vi "RT Loop - DL.vi"(11 "Message Queue":refnum<queue>) -> ()   [LabVIEW 2018]
doc: "This Control Loop VI performs control calculations of diverter line (DL) rotation."
uses:
  Support/Message Queue/Message Cluster.ctl
  Support/Message Queue/Message.ctl
  <vilib>/Platform/TimedLoop/XDataNode/timing_clust.ctl
  <vilib>/Platform/TimedLoop/XDataNode/nitl_modes.ctl
  <vilib>/Platform/TimedLoop/XDataNode/wakeup.ctl
  Controls/DL State.ctl
  <vilib>/Platform/TimedLoop/XDataNode/loadnilvce.vi
  <vilib>/Platform/TimedLoop/XDataNode/XDataNode.xnode
  <vilib>/Platform/TimedLoop/XDataNode/XDNodeRunTimeDep.lvlib
  support/Message Queue/Message Queue.lvlib
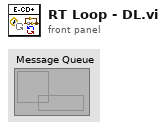
[diagram p1: front panel]
types:
  T1 = typedef "XDNodeRunTimeDep.lvlib/timing_clust.ctl" = cluster{"Expected End [f-1]":u64, "Actual End [f-1]":u64, "Finished Late? [f-1]":bool, "Expected End [i-1]":u64, "Actual End [i-1]":u64, "Finished Late? [i-1]":bool, "Expected Start [i]":u64, "Actual Start [i]":u64, "Expected Start [f]":u64, "Actual Start [f]":u64, "Source Name":string, "Structure Name":string, "Period":i64, "Deadline":i64, "Offset":i64, "Start":i64, "Priority":i32, "Timeout":i32, "Mode":T2, "Wakeup Reason":T3, "Error":errorcluster, "Source Type":string, "Secondary Source Type":string, "Global End Time":u64, "Global Start Time":u64, "Frame Duration":u64, "Iteration Duration":u64, "Assigned CPU":i32, "I/O Scan Engine Mode":u32}
  T2 = typedef "XDNodeRunTimeDep.lvlib/nitl_modes.ctl" = enum32{"No Change", "Process missed periods, maintain original phase", "Discard missed periods, maintain original phase", "Process missed periods, ignore original phase", "Discard missed periods, ignore original phase"}
  T3 = typedef "XDNodeRunTimeDep.lvlib/wakeup.ctl" = enum32{"Normal", "Aborted", "Asynchronous wakeup", "Timing source error", "Timed loop error", "Timeout"}
  T4 = typedef "DL State.ctl" = enum16{"DL STOP", "DL ROTATE CW", "DL ROTATE CCW", "SV-3 DL CW TRUE", "SV-3 DL CW FALSE", "SV-3 DL CCW TRUE", "SV-3 DL CCW FALSE"}
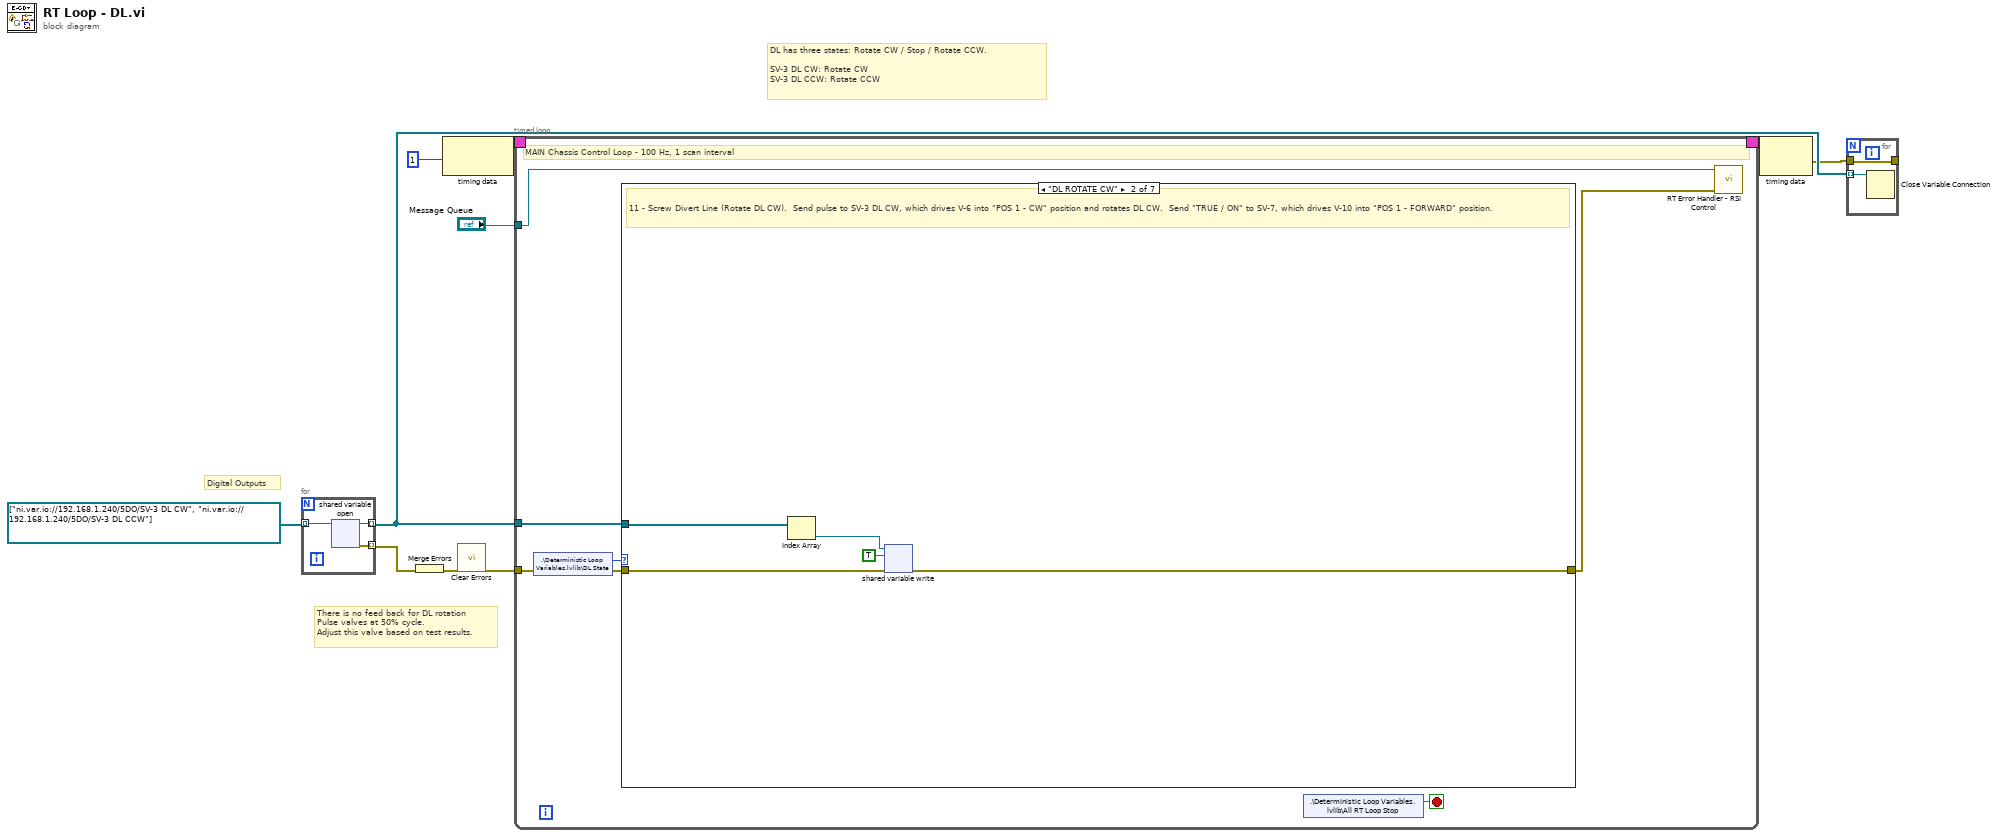
[diagram p0: block diagram]
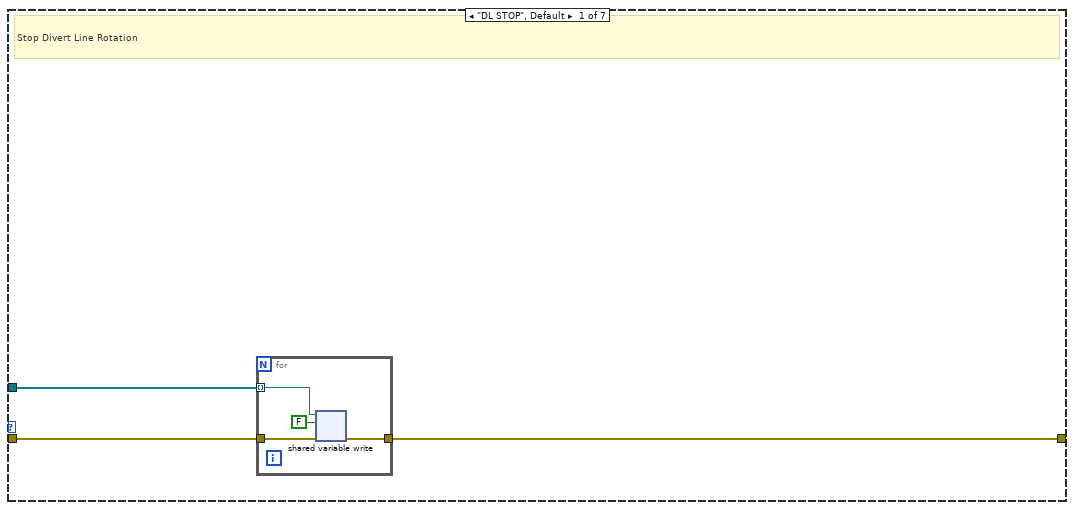
[diagram p2: hidden frame]
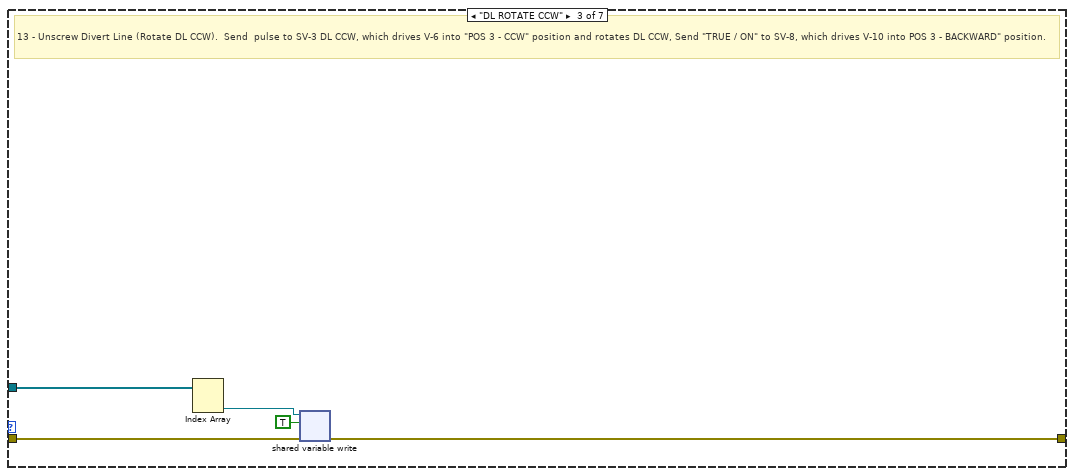
[diagram p3: hidden frame]
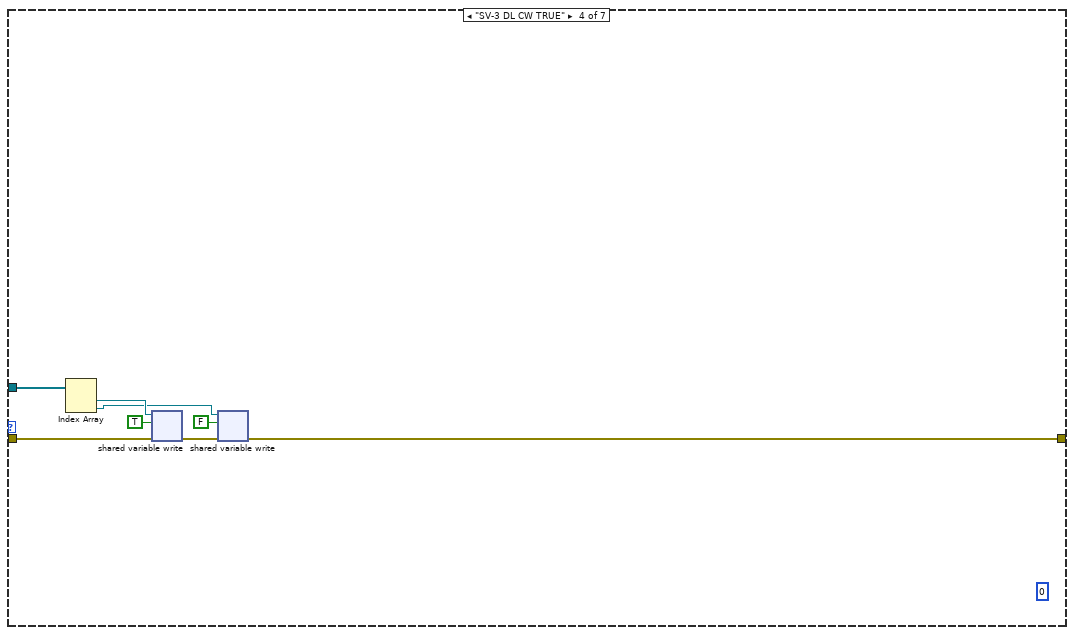
[diagram p4: hidden frame]
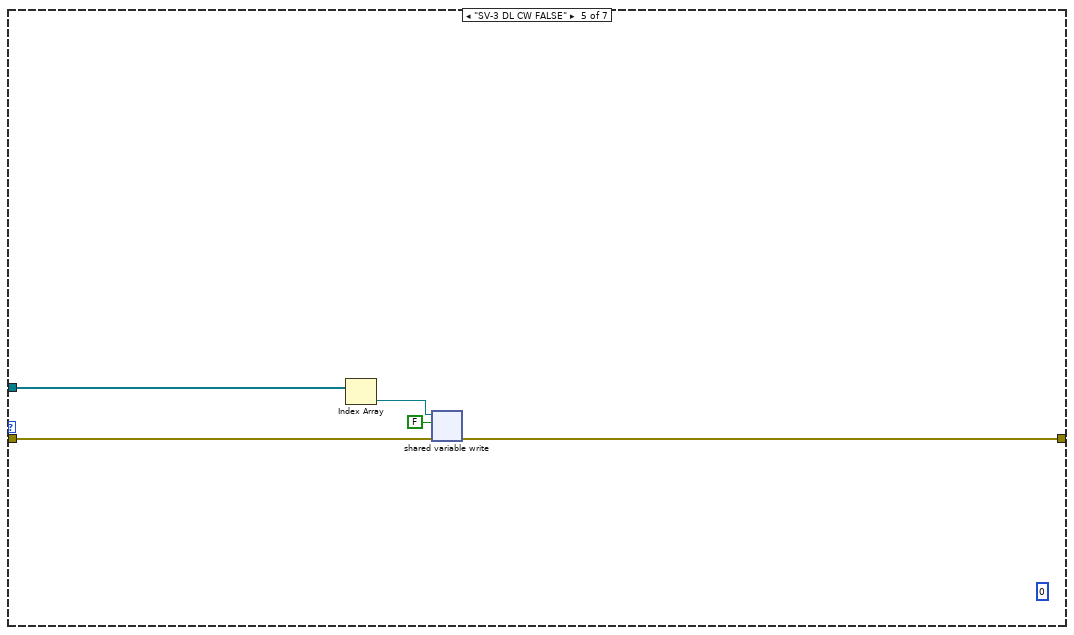
[diagram p5: hidden frame]
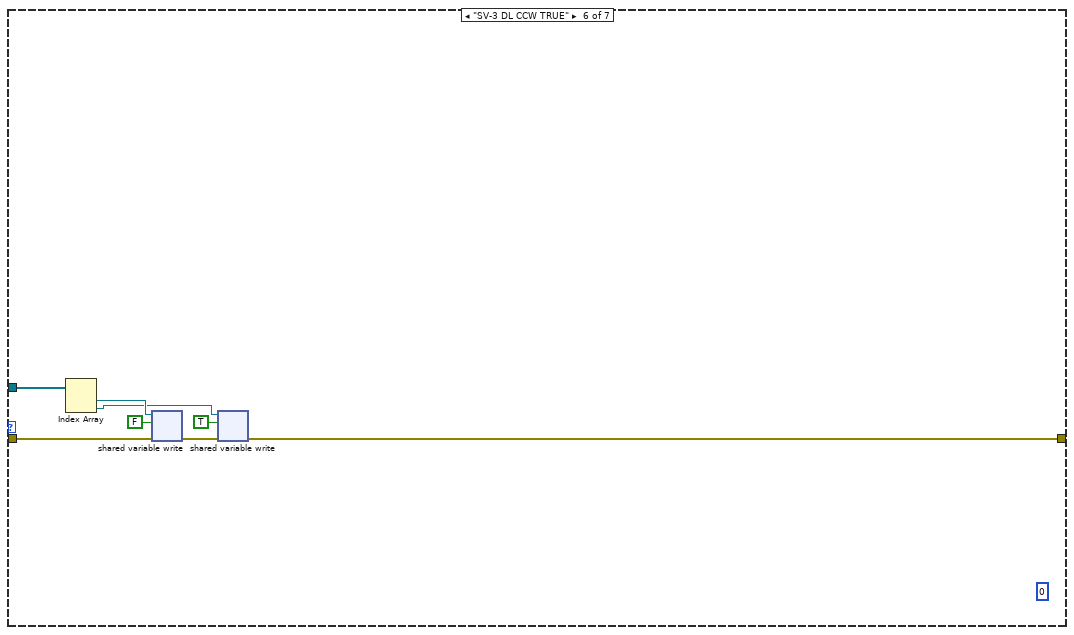
[diagram p6: hidden frame]
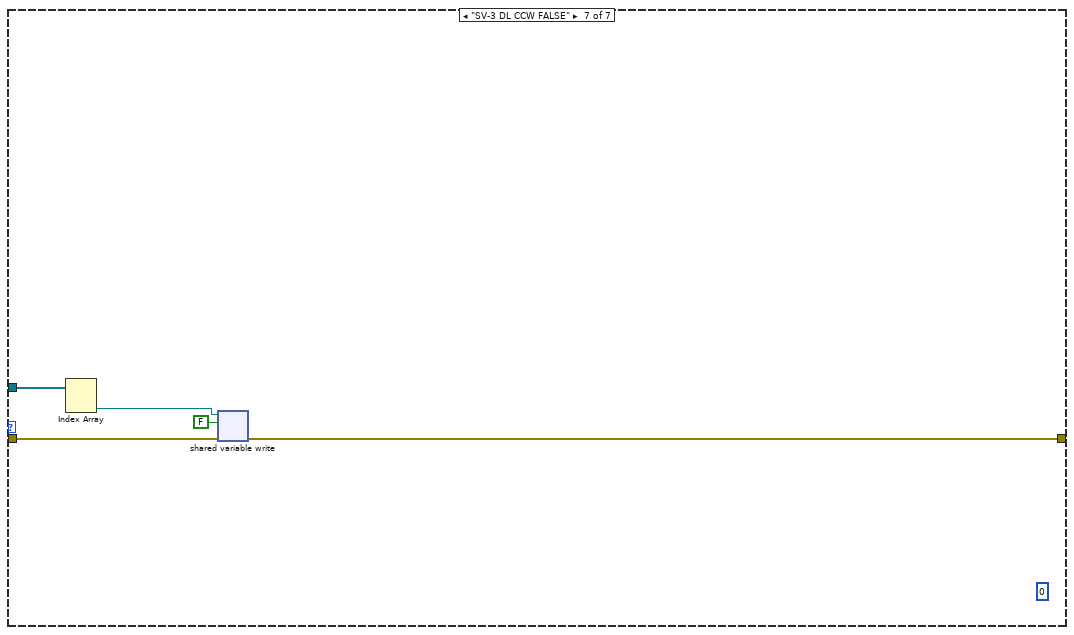
[diagram p7: hidden frame]
diagram:
  # "There is no feed back for DL rotation\nPulse valves at 50% cycle. \nAdjust this valve based on test results."
  # "Digital Outputs"
  # "DL has three states: Rotate CW / Stop / Rotate CCW.\n\nSV-3 DL CW: Rotate CW\nSV-3 DL CCW: Rotate CCW"
  n1 = for {
    tunnel: refnum<k21>[] ["ni.var.io://192.168.1.240/5DO/SV-3 DL CW", "ni.var.io://192.168.1.240/5DO/SV-3 DL CCW"] -> [w13] mode=indexing
    tunnel: [w12] -> w4 mode=indexing
    tunnel: [w11] -> w1 mode=indexing
    n2 = shared-variable-open(w13) -> (w12:refnum<k21>, w11:errorcluster)  [unwired: 1 in]
  }
  n3 = Merge Errors(w1) -> (w2:errorcluster)
  n4 = node-c288(i64 1 ("Period")) -> (w10:T1)
  n5 = call <vilib>:"Clear Errors.vi"("error in (no error)"=w2) -> ("error out"=w5:errorcluster)  [unwired: 5 in, 1 out]
  n6 = timed-loop {
    timing: w10 -> [_]
    timing-out: [_] -> w9
    tunnel: "Message Queue" -> [w15]
    tunnel: w5 -> [w17]
    tunnel: w4 -> [w19]
    stop <- w20 stop-if-true
    # "MAIN Chassis Control Loop - 100 Hz, 1 scan interval"
    n7 = shared-variable ".\\Deterministic Loop Variables.lvlib\\DL State"(error in=w17) -> (w18:T4, error out=w16:errorcluster)
    n8 = case shown="\"DL ROTATE CW\"" w18 {
      tunnel: w19 -> [w23 w31 w36 w45 w50 w58 w63]
      tunnel: w16 -> [w21 w29 w34 w42 w48 w55 w61]
      tunnel: [w22 w32 w37 w38 w47 w51 w60] -> w14
      frame "DL STOP", Default {
        # "Stop Divert Line Rotation"
        n9 = for {
          tunnel: w23 -> [w27] mode=indexing
          tunnel: w21 -> [w25]
          tunnel: [w24] -> w22
          n10 = shared-variable-write(w27, w25, FALSE ("data in")) -> (w24:errorcluster)  [unwired: 1 out]
        }
      }
      frame "DL ROTATE CW" {
        # "11 - Screw Divert Line (Rotate DL CW).  Send pulse to SV-3 DL CW, which drives V-6 into \"POS 1 - CW\" position and rotates DL CW.  Send \"TRUE / ON\" to SV-7, which drives V-10 into \"POS 1 - FORWARD\" position."
        n11 = Index Array(array=w31) -> (element=w30:refnum<k21>)  [unwired: 1 in]
        n12 = shared-variable-write(w30, w29, TRUE ("data in")) -> (w32:errorcluster)  [unwired: 1 out]
      }
      frame "DL ROTATE CCW" {
        # "13 - Unscrew Divert Line (Rotate DL CCW).  Send  pulse to SV-3 DL CCW, which drives V-6 into \"POS 3 - CCW\" position and rotates DL CCW, Send \"TRUE / ON\" to SV-8, which drives V-10 into POS 3 - BACKWARD\" position."
        n13 = Index Array(array=w36) -> (element #2=w35:refnum<k21>)  [unwired: 2 in, 1 out]
        n14 = shared-variable-write(w35, w34, TRUE ("data in")) -> (w37:errorcluster)  [unwired: 1 out]
      }
      frame "SV-3 DL CW TRUE" {
        (unwired) 0
        n15 = Index Array(array=w45) -> (element #1=w44:refnum<k21>, element #2=w43:refnum<k21>)  [unwired: 2 in]
        n16 = shared-variable-write(w44, w42, TRUE ("data in")) -> (w41:errorcluster)  [unwired: 1 out]
        n17 = shared-variable-write(w43, w41, FALSE ("data in")) -> (w38:errorcluster)  [unwired: 1 out]
      }
      frame "SV-3 DL CW FALSE" {
        (unwired) 0
        n18 = Index Array(array=w50) -> (element=w49:refnum<k21>)  [unwired: 1 in]
        n19 = shared-variable-write(w49, w48, FALSE ("data in")) -> (w47:errorcluster)  [unwired: 1 out]
      }
      frame "SV-3 DL CCW TRUE" {
        (unwired) 0
        n20 = Index Array(array=w58) -> (element #1=w57:refnum<k21>, element #2=w56:refnum<k21>)  [unwired: 2 in]
        n21 = shared-variable-write(w57, w55, FALSE ("data in")) -> (w54:errorcluster)  [unwired: 1 out]
        n22 = shared-variable-write(w56, w54, TRUE ("data in")) -> (w51:errorcluster)  [unwired: 1 out]
      }
      frame "SV-3 DL CCW FALSE" {
        (unwired) 0
        n23 = Index Array(array=w63) -> (element #2=w62:refnum<k21>)  [unwired: 2 in, 1 out]
        n24 = shared-variable-write(w62, w61, FALSE ("data in")) -> (w60:errorcluster)  [unwired: 1 out]
      }
    }
    n25 = shared-variable ".\\Deterministic Loop Variables.lvlib\\All RT Loop Stop"() -> (w20:bool)  [unwired: 1 in, 1 out]
    n26 = call "RT Error Handler - RSI Control.vi"("error in (no error)"=w14, "Message Queue"=w15) -> ()  [unwired: 8 in, 2 out]
  }
  n27 = node-c288(w9) -> (w3:errorcluster)
  n28 = for {
    tunnel: w3 -> [w66]
    tunnel: w4 -> [w67] mode=indexing
    tunnel: [w66] -> _
    n29 = Close Variable Connection(11:w67) -> ()  [unwired: 1 in, 1 out]
  }
